vi "Run Once.vi"   [LabVIEW 2014]
uses:
  2015RobotCode/Robot Global Data.vi
types:
  T1 = cluster{"normalized array[0]":dbl, "normalized array[1]":dbl, "normalized array[2]":dbl, "normalized array[3]":dbl}
  T2 = cluster{"FL Angle":dbl, "FR Angle":dbl, "RL Angle":dbl, "RR Angle":dbl}
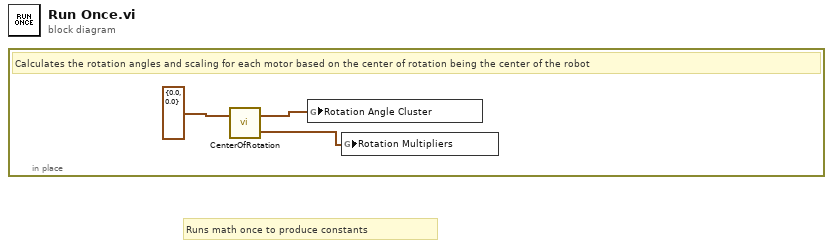
[diagram p0: block diagram]
diagram:
  # "Runs math once to produce constants"
  n1 = in-place {
    # "Calculates the rotation angles and scaling for each motor based on the center of rotation being the center of the robot"
    n2 = call "CenterOfRotation.vi"("Center of Rotation Joystick Axes"=cluster{"X":dbl, "Y":dbl} {"X"=0.0, "Y"=0.0}) -> ("Rotation Multipliers"=w1:T1, "Rotation Angle Cluster"=w2:T2)  [unwired: 1 in]
    n3 = global write "Robot Global Data.vi" "Rotation Angle Cluster"(w2) -> ()
    n4 = global write "Robot Global Data.vi" "Rotation Multipliers"(w1) -> ()
  }
